vi "Get queryserver_QueryServer_TestDataTypes Request.vi"(8 "error in (no error)":errorcluster, 11 "gRPCid in":T1) -> (0 "error out":errorcluster, 2 "Message Data":T2, 3 "gRPCid out":T1)   [LabVIEW 2019, in "TestDataMarshal.lvlib" / "TestDataMarshal.lvclass"]
uses:
  TestDataMarshal.lvclass
  gRPC lvSupport/Server API/typeDefs/grpcId.ctl
  RPC Messages/queryserver_TestDataTypesParameters/queryserver_TestDataTypesParameters_Data.ctl
  RPC Messages/queryserver_DataTypeTest/queryserver_DataTypeTest_Data.ctl
  RPC Messages/google_protobuf_Any/google_protobuf_Any_Data.ctl
  gRPC lvSupport/gprc-lvsupport.lvlib
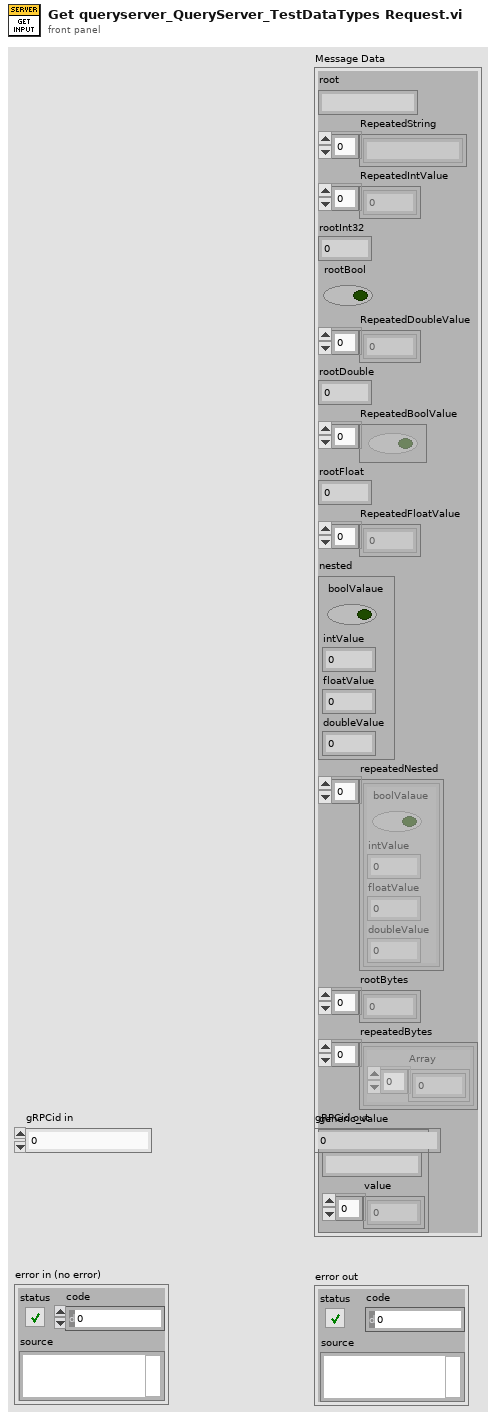
[diagram p1: front panel]
types:
  T1 = typedef "TestDataMarshal.lvlib/gprc-lvsupport.lvlib/grpcId.ctl" = u64
  T2 = typedef "TestDataMarshal.lvlib/TestDataMarshal.lvclass/queryserver_TestDataTypesParameters_Data.ctl" = cluster{"root":string, "RepeatedString":string[], "RepeatedIntValue":i32[], "rootInt32":i32, "rootBool":bool, "RepeatedDoubleValue":dbl[], "rootDouble":dbl, "RepeatedBoolValue":bool[], "rootFloat":sgl, "RepeatedFloatValue":sgl[], "nested":T3, "repeatedNested":T3[], "rootBytes":u8[], "repeatedBytes":cluster{"Array":u8[]}[], "generic_value":T4}
  T3 = typedef "TestDataMarshal.lvlib/TestDataMarshal.lvclass/queryserver_DataTypeTest_Data.ctl" = cluster{"boolValaue":bool, "intValue":i32, "floatValue":sgl, "doubleValue":dbl}
  T4 = typedef "TestDataMarshal.lvlib/TestDataMarshal.lvclass/google_protobuf_Any_Data.ctl" = cluster{"type_url":string, "value":u8[]}
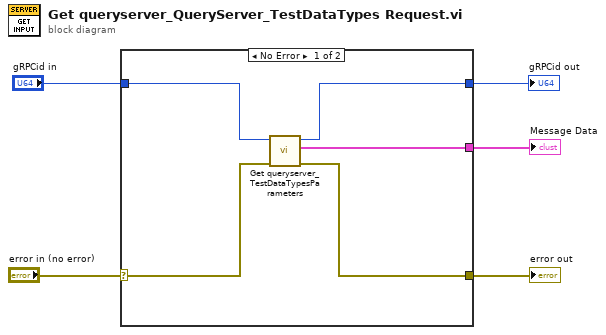
[diagram p0: block diagram]
diagram:
  n1 = case shown="No Error" "error in (no error)" {
    selector: "error in (no error)" -> [w10 w11]
    tunnel: [w9 w11] -> w4
    tunnel: "gRPCid in" -> [w8 w12]
    tunnel: [w7 _] -> w2
    tunnel: [w6 w12] -> w1
    frame No Error {
      n2 = call "Get queryserver_TestDataTypesParameters.vi"("error in (no error)"=w10, "gRPCid"=w8) -> ("error out"=w9:errorcluster, "Message Data"=w7:T2, "gRPCid out"=w6:T1)  [unwired: 7 in]
    }
    frame Error {
    }
  }
  "error out" <- w4
  "Message Data" <- w2
  "gRPCid out" <- w1
